vi "Add New MetaData Channel.vi"(8 "error in (no error)":errorcluster, 11 "Node Ptr":u64 format="%.0x") -> (0 "error out":errorcluster)   [LabVIEW 2019, in "Instrument Addon System Explorer.lvlib"]
uses:
  Instrument Addon System Explorer.lvlib
  Addon Shared/Types/MetaData Parameters.ctl
  Addon Shared/Types/Protocol Data Type.ctl
  Addon Shared/Types/Metadata Channel Type.ctl
  Addon Shared/Types/Type Cast Type.ctl
  Addon Shared/Types/Endian.ctl
  Addon Shared/SubVIs/Constants.vi
  <vilib>/NI VeriStand/Custom Device API/Custom Device API.lvlib
  Addon Shared/Instrument Addon Shared.lvlib
  APIs/Scripting API/Instrument Addon Scripting API.lvlib
panel:
  in  "Tag":string
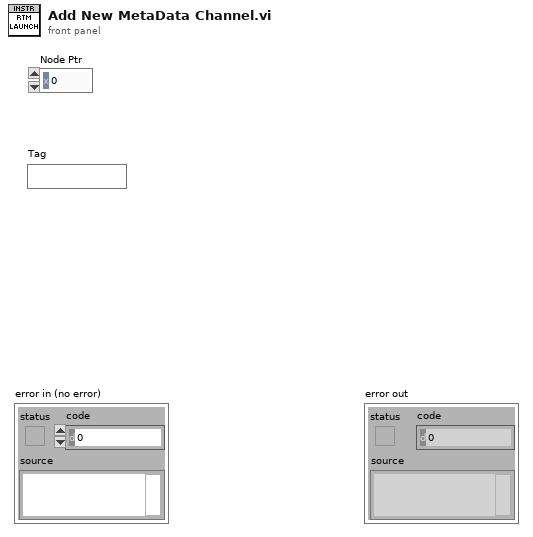
[diagram p1: front panel]
types:
  T1 = typedef "Instrument Addon Shared.lvlib/MetaData Parameters.ctl" = cluster{"Data Type":T2, "Channel Type":T3, "List":string[], "Format String":string, "Type":T4, "Delimiter":string, "Endian":T5}
  T2 = typedef "Instrument Addon Shared.lvlib/Protocol Data Type.ctl" = enum16{"Single Channel", "Array"}
  T3 = typedef "Instrument Addon Shared.lvlib/Metadata Channel Type.ctl" = enum16{"Enumerated List", "Format", "Type Cast"}
  T4 = typedef "Instrument Addon Shared.lvlib/Type Cast Type.ctl" = enum16{"DBL", "SGL", "U64", "U32", "U16", "U8", "I64", "I32", "I16", "I8"}
  T5 = typedef "Instrument Addon Shared.lvlib/Endian.ctl" = enum16{"Native", "Little", "Big"}
  T6 = typedef "Custom Device API.lvlib/Custom Device Item Info.ctl" = cluster{"Name":string, "Is Channel":bool, "GUID":string, "Is Waveform":bool}
  T7 = typedef "Custom Device API.lvlib/Custom Device Item Ref.ctl" = u64
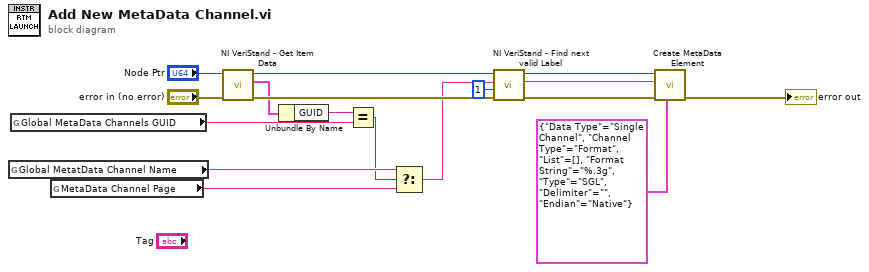
[diagram p0: block diagram]
diagram:
  n1 = global read "Constants.vi" "Global MetatData Channel Name"() -> (w10:string)
  n2 = global read "Constants.vi" "Global MetaData Channels GUID"() -> (w11:string)
  n3 = global read "Constants.vi" "MetaData Channel Page"() -> (w9:string)
  n4 = call <vilib>:"NI VeriStand - Get Item Data.vi"("error in (no error)"="error in (no error)", "Item Ref in"="Node Ptr") -> ("error out"=w16:errorcluster, "Item Info"=w13:T6, "Item Ref out"=w14:T7)  [unwired: 6 in, 1 out]
  n5 = Unbundle By Name(w13) -> ("GUID"=w12:string)
  n6 = Equal?(x=w12, y=w11) -> (x = y?=w2:bool)
  n7 = Select(t=w10, s=w2, f=w9) -> (s? t:f=w8:string)
  n8 = call <vilib>:"NI VeriStand - Find next valid Label.vi"("error in (no error)"=w16, "Start Value (1)"=1, "Label"=w8, "Item Ref in"=w14) -> ("error out"=w5:errorcluster, "Label out"=w7:string, "Item Ref out"=w6:T7)  [unwired: 3 in, 2 out]
  n9 = call "Create MetaData Element.vi"("MetaData Parameters"=T1 {"Data Type"=enum."Single Channel", "Channel Type"=enum."Format", "List"=[], "Format String"="%.3g", "Type"=enum."SGL", "Delimiter"="", "Endian"=enum."Native"}, "error in (no error)"=w5, "Name"=w7, "Refnum In"=w6) -> ("error out"=→"error out":errorcluster)  [unwired: 5 in, 2 out]
